vi "OP10_Data.vi"() -> (0 "OP10_CRIMP":T1)   [LabVIEW 2020]
panel:
  out "error out":errorcluster
  in  "error in (no error)":errorcluster
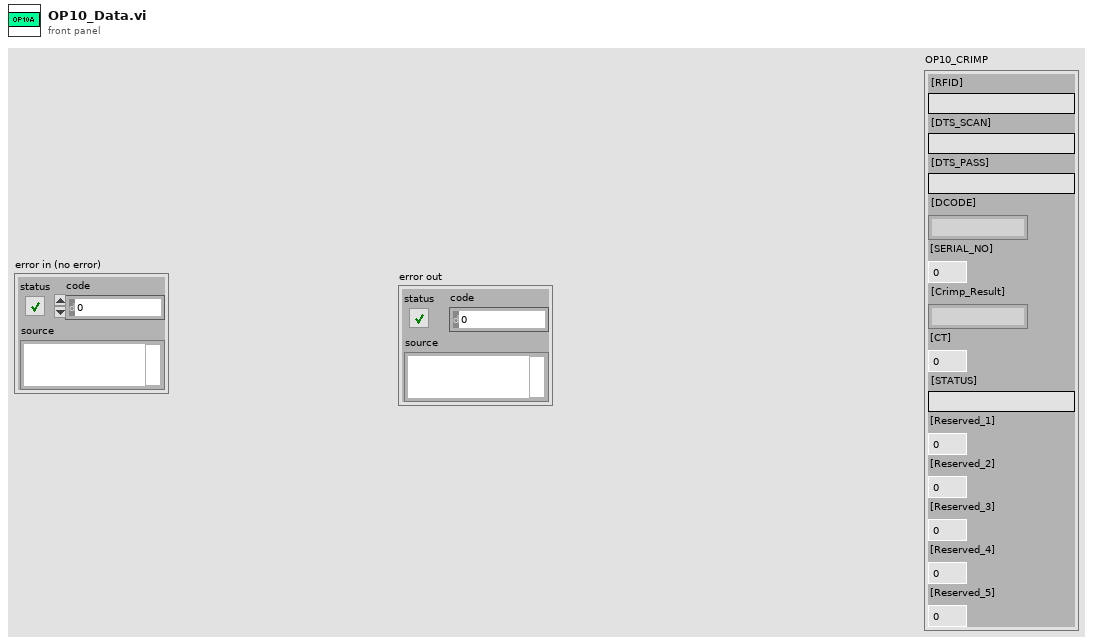
[diagram p1: front panel]
types:
  T1 = cluster{"[RFID]":string, "[DTS_SCAN]":string, "[DTS_PASS]":string, "[DCODE]":string, "[SERIAL_NO]":i32, "[Crimp_Result]":string, "[CT]":dbl, "[STATUS]":string, "[Reserved_1]":dbl, "[Reserved_2]":dbl, "[Reserved_3]":dbl, "[Reserved_4]":dbl, "[Reserved_5]":dbl}
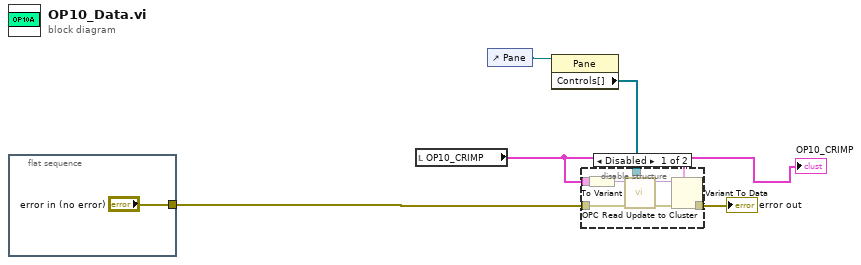
[diagram p0: block diagram]
diagram:
  n1 = flat-sequence {
    tunnel: ["error in (no error)"] -> w5
    frame #0 {
    }
  }
  n2 = local read "OP10_CRIMP"() -> (w1:T1)
  "OP10_CRIMP" <- w1
  n3 = control-ref of="Pane"() -> (w3:refnum<vi>)
  n4 = property class="Pane"(reference=w3) -> ("Controls[]"=w2:refnum<vi>[])  [unwired: 1 in, 2 out]
  n5 = disable-structure shown="Disabled" {
    disable-tunnel: w5 -> [w11 w14]
    disable-tunnel: [w9 w14] -> w4
    disable-tunnel: w2 -> [w8 _]
    disable-tunnel: w1 -> [w7 _]
    frame Disabled {
      n6 = To Variant(anything=w7) -> (Variant=w10:variant)
      n7 = call "OPC Read Update to Cluster.vi"("Controls[]"=w8, "error in (no error)"=w11, "Variant in"=w10) -> ("error out"=w12:errorcluster, "Variant out"=w13:variant)  [unwired: 7 in]
      n8 = Variant To Data(error in=w12, type=w7, Variant=w13) -> (error out=w9:errorcluster)  [unwired: 1 out]
    }
    frame Enabled {
    }
  }
  "error out" <- w4
